vi "TC.vi"() -> ()   [LabVIEW 2018]
uses:
  20181122_VI Server/20181123_VI server.llb/Global 1.vi
panel:
  in  "stop 2":bool
  in  "Open SubVI":bool
  out "current time":timestamp
  out "Numeric":dbl
  in  "Close SubVI":bool
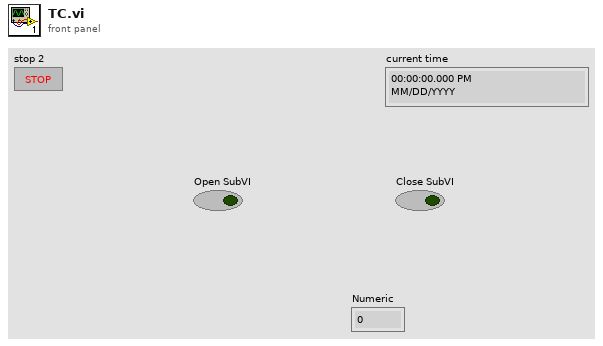
[diagram p1: front panel]
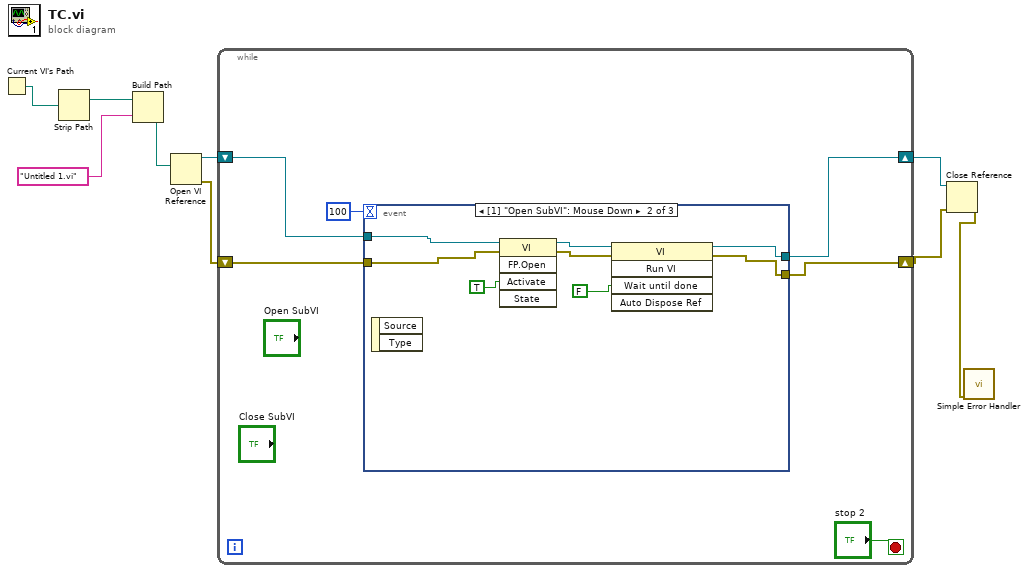
[diagram p0: block diagram]
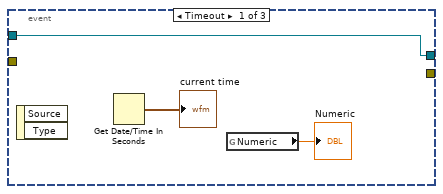
[diagram p2: hidden frame]
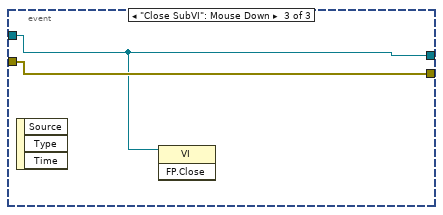
[diagram p3: hidden frame]
diagram:
  n1 = Current VI's Path() -> (path=w9:path)
  n2 = Strip Path(path=w9) -> (stripped path=w8:path)  [unwired: 1 out]
  n3 = Build Path(base path=w8, name or relative path="Untitled 1.vi") -> (appended path=w6:path)
  n4 = Open VI Reference(vi path=w6) -> (vi reference=w4:refnum<vi>, error out=w5:errorcluster)  [unwired: 5 in]
  n5 = while {
    shift-right: [w13] -> w2
    shift-left: w5 -> [w14]
    shift-right: [w10] -> w3
    shift-left: w4 -> [w11]
    stop <- "stop 2" stop-if-true
    n6 = event shown="[1] \"Open SubVI\": Mouse Down" {
      selector: _ -> [_ _ _]
      dyn-events: _ -> [_ _ _]
      timeout: 100 -> [_ _ _]
      tunnel: w14 -> [_ w20 w28]
      tunnel: [_ w22 w28] -> w13
      tunnel: w11 -> [w16 w21 w27]
      tunnel: [w16 w19 w27] -> w10
      event Timeout {
        n7 = event-data() -> ()  [unwired: 1 in, 2 out]
        n8 = Get Date/Time In Seconds() -> (seconds since 1Jan1904=→"current time":timestamp)
        n9 = global read "Global 1.vi" "Numeric"() -> (→"Numeric":dbl)
      }
      event "Open SubVI": Mouse Down {
        n10 = event-data() -> ()  [unwired: 1 in, 2 out]
        n11 = invoke class="VI" method="FP.Open"(reference=w21, error in=w20, "Activate"=TRUE ("Activate?")) -> (reference out=w24:refnum<vi>, error out=w23:errorcluster)  [unwired: 2 in, 3 out]
        n12 = invoke class="VI" method="Run VI"(reference=w24, error in=w23, "Wait until done"=FALSE ("Wait Until Done")) -> (reference out=w19:refnum<vi>, error out=w22:errorcluster)  [unwired: 2 in, 3 out]
      }
      event "Close SubVI": Mouse Down {
        n13 = event-data() -> ()  [unwired: 1 in, 3 out]
        n14 = invoke class="VI" method="FP.Close"(reference=w27) -> ()  [unwired: 2 in, 3 out]
      }
    }
  }
  n15 = Close Reference(reference=w3, error in (no error)=w2) -> (error out=w1:errorcluster)
  n16 = call <vilib>:"Simple Error Handler.vi"("error in (no error)"=w1) -> ()  [unwired: 4 in, 5 out]
